vi "Final_Cell.vi"(10 "Array in":dbl[](array[numeric]), 11 "L2T":T1) -> (0 "DeltaTcell":bool, 1 "DeltaVcell":bool, 2 "Vcell":bool[](array[boolean]), 3 "Tcell":bool[](array[boolean]))   [LabVIEW 2020]
uses:
  Ctrl/L2T.ctl
panel:
  # "Pre DCIR_____________________________________"
  # "intra DCIR_____________________________________"
  # "Post DCIR_____________________________________"
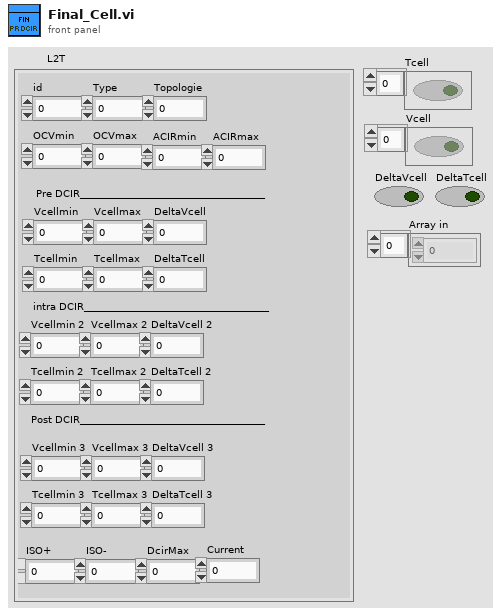
[diagram p1: front panel]
types:
  T1 = typedef "L2T.ctl" = cluster{"id":dbl, "Type":dbl, "OCVmin":dbl, "OCVmax":dbl, "ACIRmin":dbl, "ACIRmax":dbl, "Vcellmin":dbl, "Vcellmax":dbl, "DeltaVcell":dbl, "Tcellmin":dbl, "Tcellmax":dbl, "DeltaTcell":dbl, "ISO+":dbl, "ISO-":dbl, "DcirMax":dbl, "Current":dbl, "Topologie":dbl, "Vcellmin 2":dbl, "Vcellmax 2":dbl, "DeltaVcell 2":dbl, "Tcellmin 2":dbl, "Tcellmax 2":dbl, "DeltaTcell 2":dbl, "Vcellmin 3":dbl, "Vcellmax 3":dbl, "DeltaVcell 3":dbl, "Tcellmin 3":dbl, "Tcellmax 3":dbl, "DeltaTcell 3":dbl}
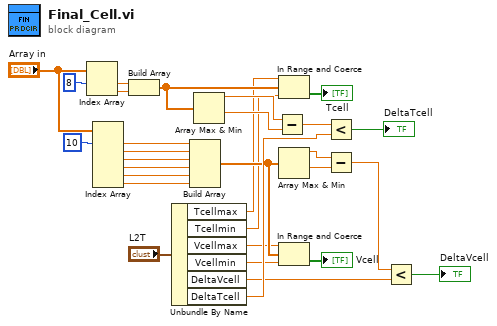
[diagram p0: block diagram]
diagram:
  n1 = Index Array(array="Array in", index #1=8 ("index")) -> (element #1=w20:dbl, element #2=w21:dbl)  [unwired: 1 in]
  n2 = Index Array(array="Array in", index #1=10 ("index")) -> (element #1=w24:dbl, element #2=w25:dbl, element #3=w26:dbl, element #4=w27:dbl, element #5=w28:dbl, element #6=w29:dbl)  [unwired: 5 in]
  n3 = Build Array(w20, w21) -> (w13:dbl[])
  n4 = Unbundle By Name("L2T") -> ("Tcellmax"=w1:dbl, "Tcellmin"=w2:dbl, "Vcellmax"=w3:dbl, "Vcellmin"=w4:dbl, "DeltaVcell"=w9:dbl, "DeltaTcell"=w14:dbl)
  n5 = Build Array(w24, w25, w26, w27, w28, w29) -> (w5:dbl[])
  n6 = Array Max & Min(array=w13) -> (max value=w10:dbl, min value=w11:dbl)  [unwired: 2 out]
  n7 = Subtract(x=w10, y=w11) -> (x-y=w12:dbl)
  n8 = In Range and Coerce ("Dans la gamme")(upper limit=w1, x=w13, lower limit=w2) -> (In Range?=→"Tcell":bool[])  [unwired: 1 out]
  n9 = Array Max & Min(array=w5) -> (max value=w6:dbl, min value=w7:dbl)  [unwired: 2 out]
  n10 = In Range and Coerce ("Dans la gamme")(upper limit=w3, x=w5, lower limit=w4) -> (In Range?=→"Vcell":bool[])  [unwired: 1 out]
  n11 = Less?(x=w12, y=w14) -> (x < y?=→"DeltaTcell":bool)
  n12 = Subtract(x=w6, y=w7) -> (x-y=w8:dbl)
  n13 = Less?(x=w8, y=w9) -> (x < y?=→"DeltaVcell":bool)
